vi "Tom_Bentham_LDA.vi"() -> (5 "Plug in titles":string[](array[string]), 7 "Plug in values":string[](array[string]))   [LabVIEW 2010]
uses:
  Globals/Plug_in_data_global.vi
  Globals/Meas_global.vi
panel:
  out "LDA 1st Comp":cluster{"Histogram of X":dbl[], "Axis":dbl[]}(graph)
  out "LDA 2nd Comp":cluster{"Histogram of X":dbl[], "Axis":dbl[]}(graph)
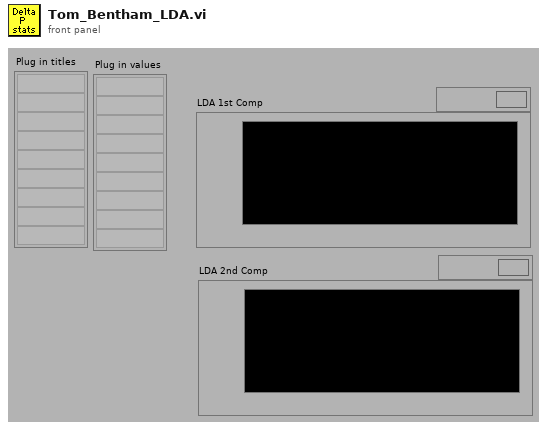
[diagram p1: front panel]
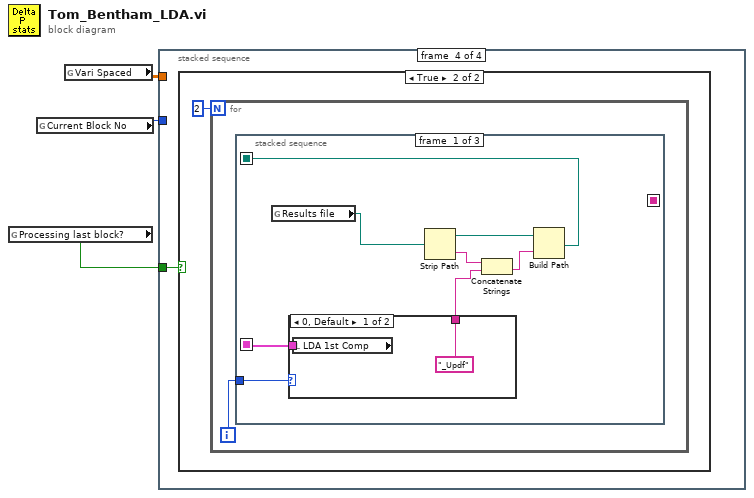
[diagram p0: block diagram]
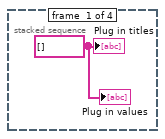
[diagram p2: hidden frame]
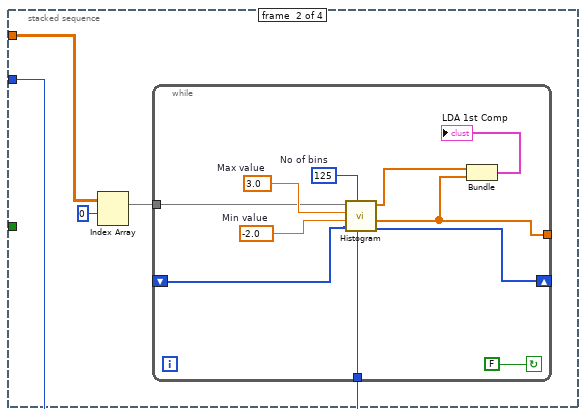
[diagram p3: hidden frame]
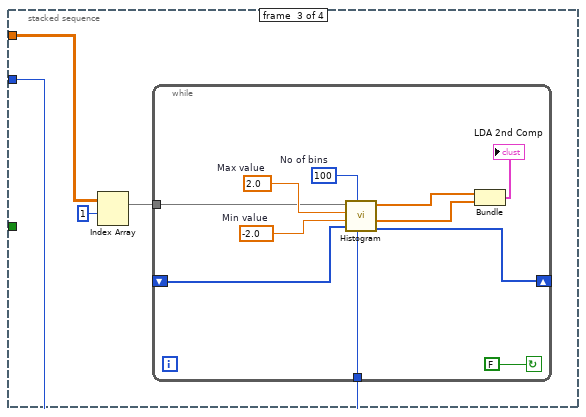
[diagram p4: hidden frame]
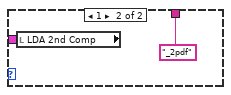
[diagram p6: hidden frame]
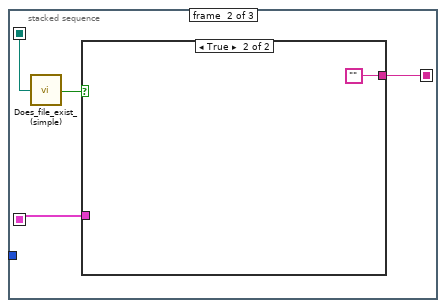
[diagram p7: hidden frame]
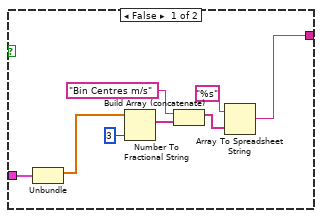
[diagram p8: hidden frame]
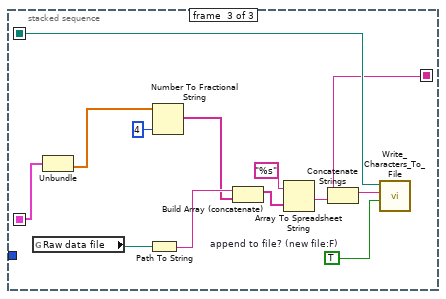
[diagram p9: hidden frame]
diagram:
  n1 = global read "Meas_global.vi" "Processing last block?"() -> (w1:bool)
  n2 = global read "Meas_global.vi" "Current Block No"() -> (w2:i32)
  n3 = global read "Plug_in_data_global.vi" "Vari Spaced"() -> (w3:dbl[][])
  n4 = stacked-sequence {
    tunnel: w3 -> [_ w6 w21 _]
    tunnel: w2 -> [_ w8 w23 _]
    tunnel: w1 -> [_ _ _ w35]
    frame #0 {
      w4 = string[] [] ("Plug in titles")
      "Plug in titles" <- w4
      "Plug in values" <- w4
    }
    frame #1 {
      n5 = Index Array(array=w6, index (row)=0) -> (element=w5:dbl[])  [unwired: 1 in]
      n6 = while {
        tunnel: w5 -> [w13]
        tunnel: w8 -> [w15]
        tunnel: [w11] -> _
        shift-left: _ -> [w14]
        shift-right: [w18] -> _
        stop <- FALSE continue-if-true
        w16 = 3.0  # Max value
        w17 = -2.0  # Min value
        w19 = 125  # No of bins
        n7 = call "Histogram.vi"("Current Block No"=w15, "No of bins"=w19, "Shift Hist"=w14, "Min value"=w17, "Max value"=w16, "X"=w13) -> ("Shift Hist"=w18:i32[], "Histogram of X"=w11:dbl[], "Axis"=w12:dbl[])  [unwired: 2 in]
        n8 = Bundle("Axis"=w12, "Histogram of X"=w11) -> (→"LDA 1st Comp":cluster{"Axis":dbl[], "Histogram of X":dbl[]})  [unwired: 1 in]
      }
    }
    frame #2 {
      n9 = Index Array(array=w21, index (row)=1) -> (element=w20:dbl[])  [unwired: 1 in]
      n10 = while {
        tunnel: w20 -> [w28]
        tunnel: w23 -> [w30]
        shift-left: _ -> [w29]
        shift-right: [w33] -> _
        stop <- FALSE continue-if-true
        w31 = 2.0  # Max value
        w32 = -2.0  # Min value
        w34 = 100  # No of bins
        n11 = call "Histogram.vi"("Current Block No"=w30, "No of bins"=w34, "Shift Hist"=w29, "Min value"=w32, "Max value"=w31, "X"=w28) -> ("Shift Hist"=w33:i32[], "Histogram of X"=w25:dbl[], "Axis"=w26:dbl[])  [unwired: 2 in]
        n12 = Bundle("Axis"=w26, "Histogram of X"=w25) -> (→"LDA 2nd Comp":cluster{"Axis":dbl[], "Histogram of X":dbl[]})  [unwired: 1 in]
      }
    }
    frame #3 {
      n13 = case shown="True" w35 {
        frame False {
        }
        frame True {
          n14 = for {
            N: 2 -> [_]
            i -> [w37]
            n15 = stacked-sequence {
              seq-local: [w40 _ _] -> [_ w51 w68]
              seq-local: [w39 _ _] -> [_ w53 w67]
              seq-local: [_ w50 _] -> [_ _ w64]
              tunnel: w37 -> [w42 _ _]
              frame #0 {
                n16 = global read "Meas_global.vi" "Results file"() -> (w38:path)
                n17 = case shown="0, Default" w42 {
                  tunnel: ["_Updf" ("Substring") "_2pdf" ("Substring")] -> w41
                  tunnel: [w46 w48] -> w40
                  frame 0, Default {
                    n18 = local read "LDA 1st Comp"() -> (w46:cluster{"Histogram of X":dbl[], "Axis":dbl[]})
                  }
                  frame 1 {
                    n19 = local read "LDA 2nd Comp"() -> (w48:cluster{"Histogram of X":dbl[], "Axis":dbl[]})
                  }
                }
                n20 = Strip Path(path=w38) -> (stripped path=w45:path, name=w44:string)
                n21 = Concatenate Strings(w44, w41) -> (w43:string)
                n22 = Build Path(base path=w45, name or relative path=w43) -> (appended path=w39:path)
              }
              frame #1 {
                n23 = call "Does_file_exist_(simple).vi"("Pathname"=w53) -> ("exists?"=w52:bool)
                n24 = case shown="True" w52 {
                  tunnel: w51 -> [w61 _]
                  tunnel: [w54 ""] -> w50
                  frame False {
                    n25 = Unbundle(w61) -> ("Histogram of X"=w59:dbl[])  [unwired: 1 out]
                    n26 = Number To Fractional String(number=w59, precision (6)=i16 3) -> (F-format string=w56:string[])  [unwired: 2 in]
                    n27 = Build Array (concatenate)("Bin Centres m/s" ("Input Element"), w56) -> (w58:string[])
                    n28 = Array To Spreadsheet String(array=w58, 3:"%s" ("format string")) -> (spreadsheet string=w54:string)  [unwired: 1 in]
                  }
                  frame True {
                  }
                }
              }
              frame #2 {
                w69 = TRUE  # append to file? (new file:F)
                n29 = global read "Meas_global.vi" "Raw data file"() -> (w74:path)
                n30 = Unbundle(w68) -> ("Axis"=w66:dbl[])  [unwired: 1 out]
                n31 = Path To String(path=w74) -> (string=w73:string)
                n32 = Number To Fractional String(number=w66, precision (6)=i16 4) -> (F-format string=w72:string[])  [unwired: 2 in]
                n33 = Build Array (concatenate)(w73, w72) -> (w71:string[])
                n34 = Array To Spreadsheet String(array=w71, 3:"%s" ("format string")) -> (spreadsheet string=w65:string)  [unwired: 1 in]
                n35 = Concatenate Strings(w64, w65) -> (w63:string)
                n36 = call "Write_Characters_To_File.vi"("file path (dialog if empty)"=w67, "character string"=w63, "append to file? (new file:F)"=w69) -> ()  [unwired: 5 in, 1 out]
              }
            }
          }
        }
      }
    }
  }
